vi "Login.vi"() -> ()   [LabVIEW 2020]
uses:
  Global.vi
panel:
  in  "密码":string
  in  "账号":string
  in  "确定":bool
  # "C-EPS生产质量追溯系统"
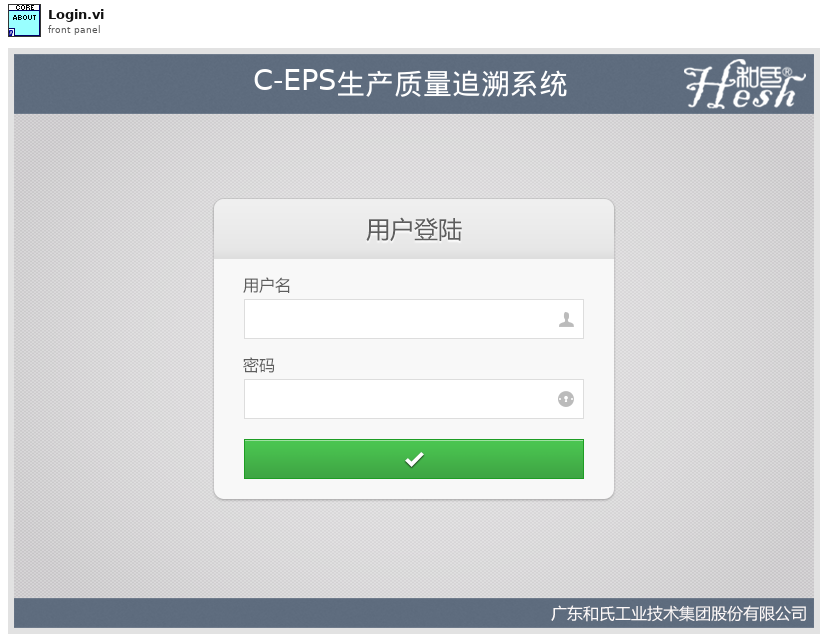
[diagram p1: front panel]
types:
  T1 = enum32{"Invalid", "Standard", "Closed", "Hidden", "Minimized", "Maximized"}
  T2 = cluster{"data[0]":string, "data[1]":string, "data[2]":string, "data[3]":string}
  T3 = typedef "eventvkey.ctl" = enum16{"ASCII", "Enter", "Return", "Shift", "Ctrl", "Alt", "Cmd", "Opt", "Caps", "NumLock", "Clear", "Break", "Up", "Down", "Left", "Right", "Insert", "Delete", "Home", "End", "PageUp", "PageDown", "Escape", "Help", "Pause", "ScrollLock", "F1", "F2", "F3", "F4", "F5", "F6", "F7", "F8", "F9", "F10", "F11", "F12", "F13", "F14", "F15", "F16", "F17", "F18", "F19", "F20", "F21", "F22", "F23", "F24", "Play", "VolumeUp", "VolumeDown", "Mute", "Two Byte Char"}
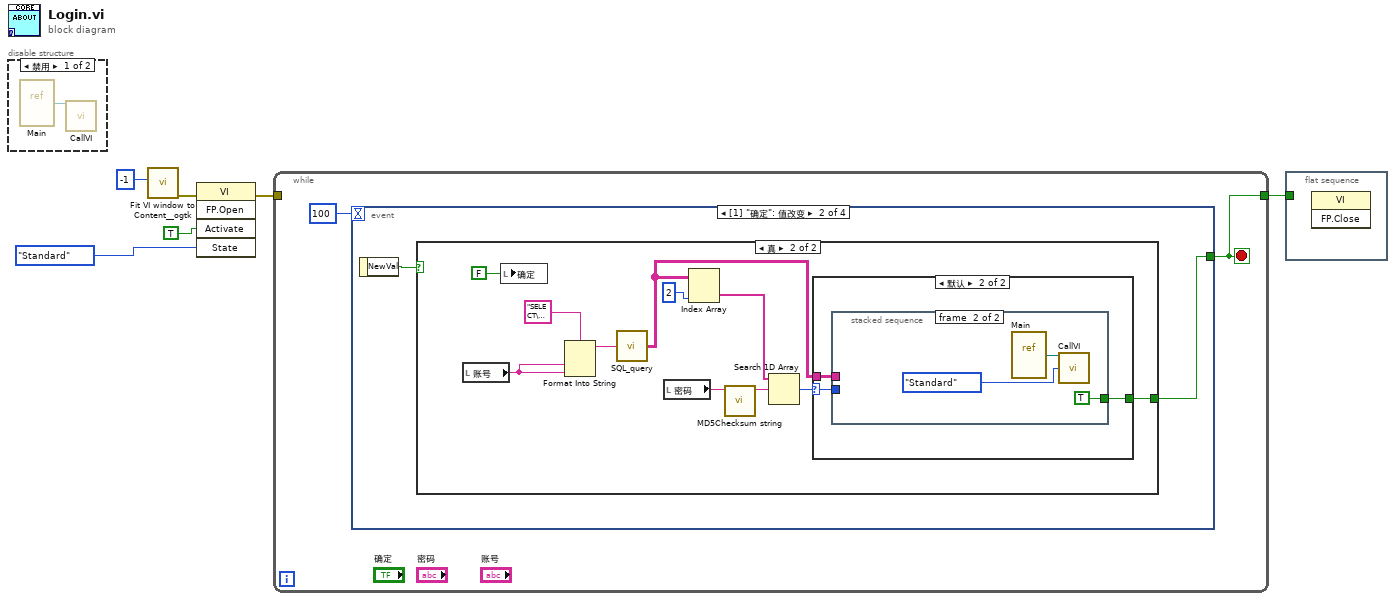
[diagram p0: block diagram]
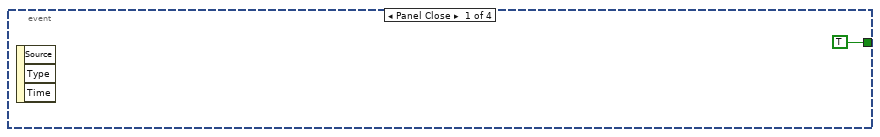
[diagram p3: hidden frame]
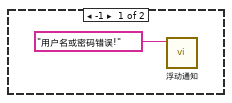
[diagram p5: hidden frame]
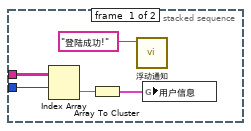
[diagram p6: hidden frame]
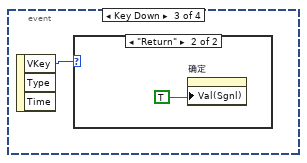
[diagram p7: hidden frame]
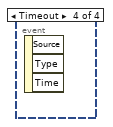
[diagram p9: hidden frame]
diagram:
  n1 = disable-structure shown="禁用" {
    frame Disabled {
      n2 = vi-ref "Main.vi"() -> (w7:refnum<vi>)
      n3 = call "CallVI.vi"("VI引用"=w7) -> ()  [unwired: 12 in, 3 out]
    }
    frame Enabled {
    }
  }
  n4 = call <userlib>:"Fit VI window to Content__ogtk.vi"("border spacing (2 px)"=-1) -> ("error out"=w2:errorcluster)  [unwired: 5 in, 1 out]
  n5 = invoke class="VI" method="FP.Open"(error in=w2, "Activate"=TRUE ("Activate?"), "State"=T1."Standard") -> (error out=w1:errorcluster)  [unwired: 2 in, 4 out]
  n6 = while {
    tunnel: [w9] -> w6
    tunnel: w1 -> [_]
    stop <- w9 stop-if-true
    n7 = event shown="[1] \"确定\": 值改变" {
      selector: _ -> [_ _ _ _]
      dyn-events: _ -> [_ _ _ _]
      timeout: 100 -> [_ _ _ _]
      tunnel: [TRUE w11 _ _] -> w9
      event Panel Close {
        n8 = event-data() -> ()  [unwired: 4 out]
      }
      event "确定": Value Change {
        n9 = event-data() -> ("NewVal"=w12:bool)  [unwired: 1 out]
        n10 = case shown="真" w12 {
          tunnel: [_ w14] -> w11
          frame False {
          }
          frame True {
            n11 = local read "账号"() -> (w20:string)
            n12 = local write "确定"(FALSE ("确定")) -> ()
            n13 = Format Into String(format string="SELECT\ndbo.[User].USER_EMPLOYEE_ID,\ndbo.[User].USER_NAME,\ndbo.[User].USER_PASSWD,\ndbo.[User].USER_PERMIT\n\nFROM\ndbo.[User]\nWHERE\ndbo.[User].USER_NAME = '%s' \nOR\ndbo.[User].USER_EMPLOYEE_ID = '%s'\n" ("格式字符串"), w20, w20) -> (resulting string=w17:string)  [unwired: 2 in, 1 out]
            n14 = call "SQL_query.vi"("SQL query"=w17) -> ("data"=w15:string[][])  [unwired: 3 in, 1 out]
            n15 = local read "密码"() -> (w21:string)
            n16 = Index Array(array=w15, index (col)=2 ("禁用的索引 (列)")) -> (element=w19:string[])  [unwired: 1 in]
            n17 = call <vilib>:"MD5Checksum string.vi"("Message String"=w21) -> ("MD5 message-digest"=w22:string)  [unwired: 10 in]
            n18 = Search 1D Array(1D array=w19, element=w22) -> (index of element=w16:i32)  [unwired: 1 in]
            n19 = case shown="默认" w16 {
              selector: w16 -> [_ w26]
              tunnel: w15 -> [_ w27]
              tunnel: [_ w25] -> w14
              frame -1 {
                n20 = call "浮动通知.vi"("通知内容"="用户名或密码错误!") -> ()  [unwired: 11 in]
              }
              frame Default {
                n21 = stacked-sequence {
                  tunnel: w27 -> [w32 _]
                  tunnel: w26 -> [w31 _]
                  tunnel: [_ TRUE] -> w25
                  frame #0 {
                    n22 = Index Array(array=w32, index (row)=w31) -> (element=w29:string[])  [unwired: 1 in]
                    n23 = Array To Cluster(array=w29) -> (cluster=w28:T2)
                    n24 = call "浮动通知.vi"("通知内容"="登陆成功!") -> ()  [unwired: 11 in]
                    n25 = global write "Global.vi" "用户信息"(w28) -> ()
                  }
                  frame #1 {
                    n26 = vi-ref "Main.vi"() -> (w34:refnum<vi>)
                    n27 = call "CallVI.vi"("VI引用"=w34, "状态"=T1."Standard") -> ()  [unwired: 11 in, 3 out]
                  }
                }
              }
            }
          }
        }
      }
      event Key Down {
        n28 = event-data() -> ("VKey"=w36:T3)  [unwired: 3 out]
        n29 = case shown="\"Return\"" w36 {
          frame Default {
          }
          frame "Return" {
            n30 = property on="确定" class="Bool (严格)"("Val(Sgnl)"=TRUE ("值(信号)")) -> ()  [unwired: 2 in, 2 out]
          }
        }
      }
      event Timeout {
        n31 = event-data() -> ()  [unwired: 4 out]
      }
    }
  }
  n32 = flat-sequence {
    tunnel: w6 -> [_]
    frame #0 {
      n33 = invoke class="VI" method="FP.Close"() -> ()  [unwired: 3 in, 3 out]
    }
  }
